vi "getAll.vi"(8 "error in (no error)":errorcluster, 11 "instrument.PPMS in":refnum<class "instrument.PPMS.lvclass">) -> (0 "error out":errorcluster, 2 "getAll":variant, 3 "instrument.PPMS out":refnum<class "instrument.PPMS.lvclass">)   [LabVIEW 2020, in "instrument.PPMS.lvclass"]
uses:
  instrument.PPMS.lvclass
  Typedefs/PPMS.getAll--cluster.ctl
  Typedefs/PPMS.Temperature Status--ring.ctl
  Typedefs/PPMS.Magnet Status--ring.ctl
  instrument.PPMS.lvclass/instrument.PPMS.ctl
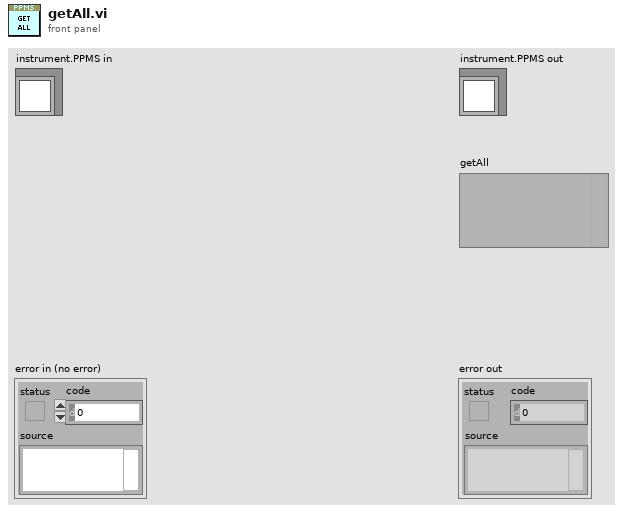
[diagram p1: front panel]
types:
  T1 = typedef "instrument.PPMS.lvclass/PPMS.getAll--cluster.ctl" = cluster{"PPMS 1 Helium Level":dbl, "PPMS 1 Temperature":dbl, "PPMS 1 Temperature Status":T2, "PPMS 1 Magnetic Field":dbl, "PPMS 1 Magnet Status":T3}
  T2 = typedef "instrument.PPMS.lvclass/PPMS.Temperature Status--ring.ctl" = i32
  T3 = typedef "instrument.PPMS.lvclass/PPMS.Magnet Status--ring.ctl" = i32
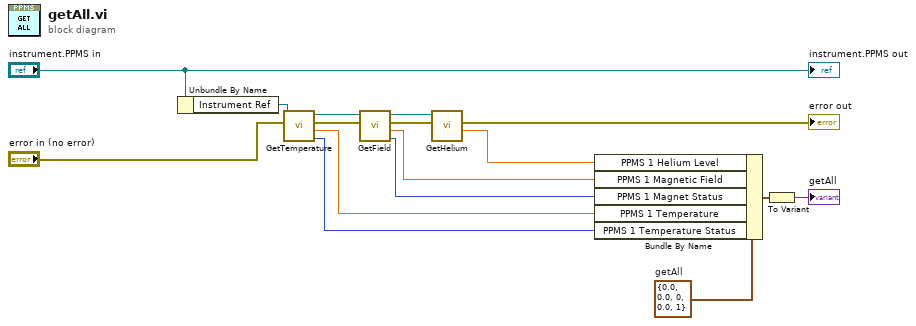
[diagram p0: block diagram]
diagram:
  w14 = T1 {"PPMS 1 Helium Level"=0.0, "PPMS 1 Temperature"=0.0, "PPMS 1 Temperature Status"=0, "PPMS 1 Magnetic Field"=0.0, "PPMS 1 Magnet Status"=1}  # getAll
  n1 = Unbundle By Name("instrument.PPMS in") -> ("Instrument Ref"=w10:refnum<k24>)
  n2 = call "GetTemperature.vi"("error in (no error)"="error in (no error)", "Instrument Ref In"=w10) -> ("Temperature\nStatus"=w5:i32, "Temperature"=w12:dbl, "error out"=w16:errorcluster, "Instrument Ref Out"=w15:refnum<k24>)  [unwired: 3 in, 1 out]
  n3 = call "GetField.vi"("error in (no error)"=w16, "Instrument Ref In"=w15) -> ("Field\nStatus"=w6:i32, "Field"=w13:dbl, "error out"=w4:errorcluster, "Instrument Ref Out"=w3:refnum<k24>)  [unwired: 3 in, 1 out]
  n4 = call "GetHelium.vi"("error in (no error)"=w4, "Instrument Refnum in"=w3) -> ("Helium Level (%)"=w1:dbl, "error out"=→"error out":errorcluster)  [unwired: 3 in, 1 out]
  n5 = Bundle By Name(cluster=w14, "PPMS 1 Helium Level"=w1, "PPMS 1 Magnetic Field"=w13, "PPMS 1 Magnet Status"=w6, "PPMS 1 Temperature"=w12, "PPMS 1 Temperature Status"=w5) -> (w7:T1)
  n6 = To Variant(anything=w7) -> (Variant=→"getAll":variant)
  "instrument.PPMS out" <- "instrument.PPMS in"
